vi "PSFLSHdll_d.vi"(5 "dll_path_in":path, 8 "error in (no error)":errorcluster, 9 "Component Molar Fractions":dbl[](array[numeric])=[1.0, 0.0, 0.0, 0.0, 0.0, 0.0, 0.0, 0.0, 0.0, 0.0, 0.0, 0.0, 0.0, 0.0, 0.0, 0.0, 0.0, 0.0, 0.0, 0.0], 10 "p":dbl, 11 "S":dbl=30.0) -> (0 "error out":errorcluster, 3 "psdataout":dbl[](array[numeric]), 4 "dll_path_out":path)   [LabVIEW 2017]
doc: "Please feel free to contact me if you have any questions .\nMy mail:ken_pop@tom.com yan.ding@jci.com"
panel:
  out "x":dbl[](array[numeric])
  out "d":dbl
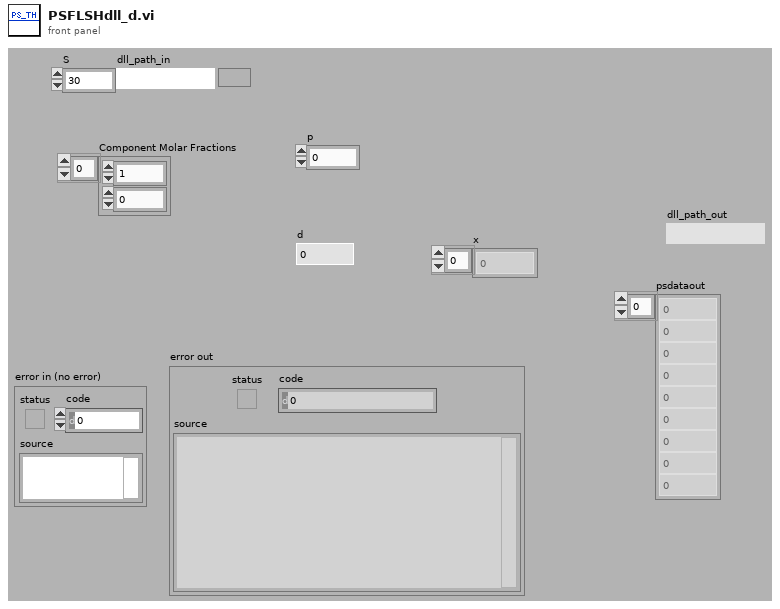
[diagram p1: front panel]
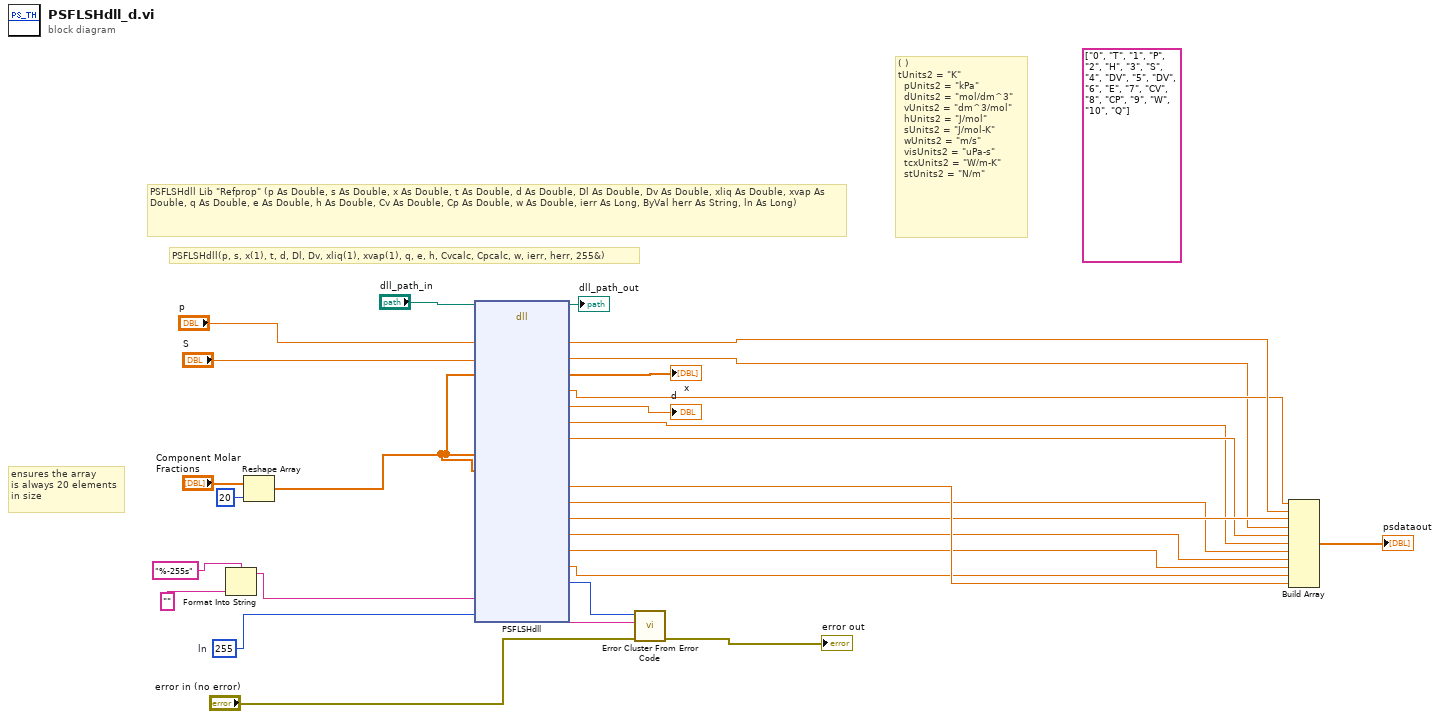
[diagram p0: block diagram]
diagram:
  (unwired) string[][] [["0", "T"], ["1", "P"], ["2", "H"], ["3", "S"], ["4", "DV"], ["5", "DV"], ["6", "E"], ["7", "CV"], ["8", "CP"], ["9", "W"], ["10", "Q"]]
  w21 = 255  # ln
  # "( )\ntUnits2 = \"K\"\n  pUnits2 = \"kPa\"\n  dUnits2 = \"mol/dm^3\"\n  vUnits2 = \"dm^3/mol\"\n  hUnits2 = \"J/mol\"\n  sUnits2 = \"J/mol-K\"\n  wUnits2 = \"m/s\"\n  visUnits2 = \"uPa-s\"\n  tcxUnits2 = \"W/m-K\"\n  stUnits2 = \"N/m\""
  # "PSFLSHdll Lib \"Refprop\" (p As Double, s As Double, x As Double, t As Double, d As Double, Dl As Double, Dv As Double, xliq As Double, xvap As Double, q As Double, e As Double, h As Double, Cv As Double, Cp As Double, w As Double, ierr As Long, ByVal herr As String, ln As Long)"
  # "PSFLSHdll(p, s, x(1), t, d, Dl, Dv, xliq(1), xvap(1), q, e, h, Cvcalc, Cpcalc, w, ierr, herr, 255&)"
  # "ensures the array\nis always 20 elements\nin size"
  n1 = Format Into String(format string="%-255s", "") -> (resulting string=w20:string)  [unwired: 2 in, 1 out]
  n2 = Reshape Array("Component Molar Fractions", 20 ("dimension size")) -> (w18:dbl[])
  n3 = dll-call lib="refprop.DLL" fn="PSFLSHdll"(path in="dll_path_in", "p"="p", "s"="S", "x"=w18, "xliq"=w18, "xvap"=w18, "herr"=w20, "ln"=w21) -> (path out=→"dll_path_out":path, "p"=w13:dbl, "s"=w9:dbl, "x"=→"x":dbl[], "t"=w11:dbl, "d"=→"d":dbl, "Dl"=w7:dbl, "Dv"=w8:dbl, "q"=w12:dbl, "e"=w6:dbl, "h"=w10:dbl, "cv"=w5:dbl, "cp"=w4:dbl, "w"=w3:dbl, "ierr"=w22:i32, "herr"=w23:string)  [unwired: 17 in, 1 out]
  n4 = call <vilib>:"Error Cluster From Error Code.vi"("error in (no error)"="error in (no error)", "error message (\"\")"=w23, "error code (0)"=w22) -> ("error out"=→"error out":errorcluster)  [unwired: 6 in]
  n5 = Build Array(w11, w13, w10, w9, w8, w7, w6, w5, w4, w3, w12) -> (→"psdataout":dbl[])
